vi "Error Bar Plot.vi"() -> ()   [LabVIEW 2020]
doc: "This VI shows how to use the Error Bar Plot indicator."
uses:
  <vilib>/Math Plots/2D Math Plots/2D Error Bar/2D Error Bar XCtrl/2D Error Bar.xctl
  <vilib>/Math Plots/2D Math Plots/2D Error Bar/2D Error Bar Datatype/Public/Plot Helper (Percentage).vi
  <vilib>/Math Plots/2D Math Plots/2D Error Bar/2D Error Bar Datatype/2D Error Bar Datatype.lvclass
panel:
  out "Error Bar Plot":refnum<class "2D Plot Datatype.lvclass">[](xcontrol)
  # "Overview: Demonstrates the Error Bar Plot indicator.\nInstructions:\nRun the VI."
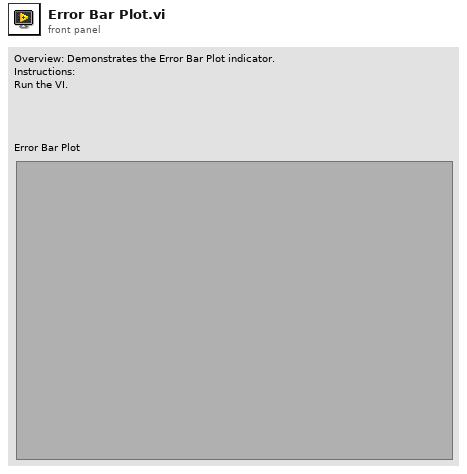
[diagram p1: front panel]
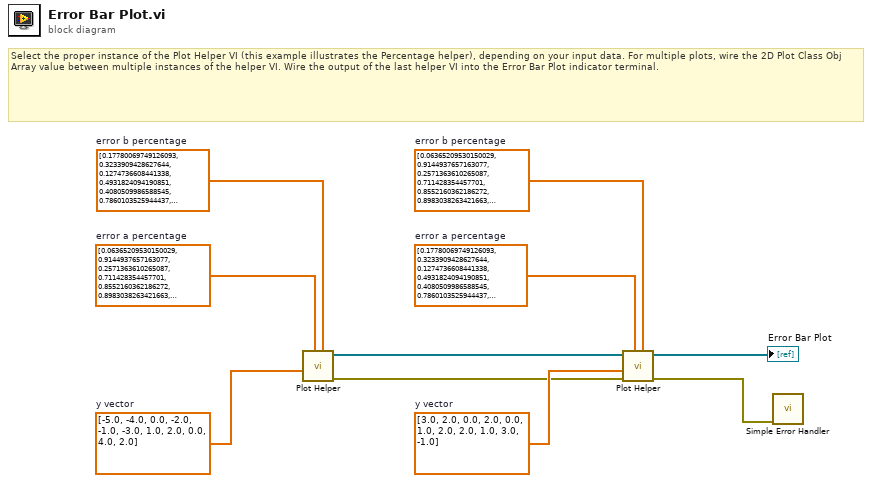
[diagram p0: block diagram]
diagram:
  w5 = dbl[] [0.06365209530150029, 0.9144937657163077, 0.2571363610265087, 0.711428354457701, 0.8552160362186272, 0.8983038263421663, 0.7981564262749408, 0.8357268761166425, 0.9137256426233773, 0.16585971651054843, 0.054870619396038656]  # error b percentage
  w4 = dbl[] [0.17780069749126093, 0.3233909428627644, 0.1274736608441338, 0.4931824094190851, 0.4080509986588545, 0.7860103525944437, 0.9479983309200797, 0.23832769134275944, 0.15590700978639616, 0.9730896860955609, 0.7101179345115022]  # error a percentage
  w6 = dbl[] [0.17780069749126093, 0.3233909428627644, 0.1274736608441338, 0.4931824094190851, 0.4080509986588545, 0.7860103525944437, 0.9479983309200797, 0.23832769134275944, 0.15590700978639616, 0.9730896860955609, 0.7101179345115022]  # error b percentage
  w7 = dbl[] [3.0, 2.0, 0.0, 2.0, 0.0, 1.0, 2.0, 2.0, 1.0, 3.0, -1.0]  # y vector
  w10 = dbl[] [-5.0, -4.0, 0.0, -2.0, -1.0, -3.0, 1.0, 2.0, 0.0, 4.0, 2.0]  # y vector
  w9 = dbl[] [0.06365209530150029, 0.9144937657163077, 0.2571363610265087, 0.711428354457701, 0.8552160362186272, 0.8983038263421663, 0.7981564262749408, 0.8357268761166425, 0.9137256426233773, 0.16585971651054843, 0.054870619396038656]  # error a percentage
  # "Select the proper instance of the Plot Helper VI (this example illustrates the Percentage helper), depending on your input data. For multiple plots, wire the 2D Plot Class Obj Array value between multiple instances of the helper VI. Wire the output of the last helper VI into the Error Bar Plot indicator terminal."
  n1 = call-poly <vilib>:"Plot Helper.vi"("error b percentage"=w6, "error a percentage"=w9, "y vector"=w10) -> ("error out"=w2:errorcluster, "2D Plot Class Obj Array out"=w8:refnum<class "2D Plot Datatype.lvclass">[])  [unwired: 3 in, 4 out]
  n2 = call-poly <vilib>:"Plot Helper.vi"("error b percentage"=w5, "error a percentage"=w4, "error in (no error)"=w2, "y vector"=w7, "2D Plot Class Obj Array in"=w8) -> ("error out"=w1:errorcluster, "2D Plot Class Obj Array out"=→"Error Bar Plot":refnum<class "2D Plot Datatype.lvclass">[])  [unwired: 1 in, 4 out]
  n3 = call <vilib>:"Simple Error Handler.vi"("error in (no error)"=w1) -> ()  [unwired: 4 in, 5 out]
